vi "LVIS_FilePosition.vi"(8 "Error In":errorcluster, 9 "Action":enum16{"Read", "Write", "Set"}(ring), 10 "Position In":i32, 11 "Ref In":refnum<file>) -> (0 "Error out":errorcluster, 2 "Position Out":i32, 3 "Ref Out":refnum<file>)   [LabVIEW 2015]
doc: "Reads, writes and sets the current backup file position based on the LVIS_Setting FilePosition value."
uses:
  Globals/LVIS_IsGlobal.vi
  <vilib>/Utility/config.llb/Read Key (String).vi
  <vilib>/Utility/config.llb/Write Key (String).vi
  <vilib>/Utility/config.llb/NI_LVConfig.lvlib
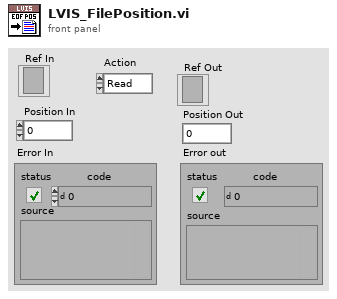
[diagram p1: front panel]
types:
  T1 = typedef "NI_LVConfig.lvlib/Config Data RefNum.ctl" = refnum<k1>
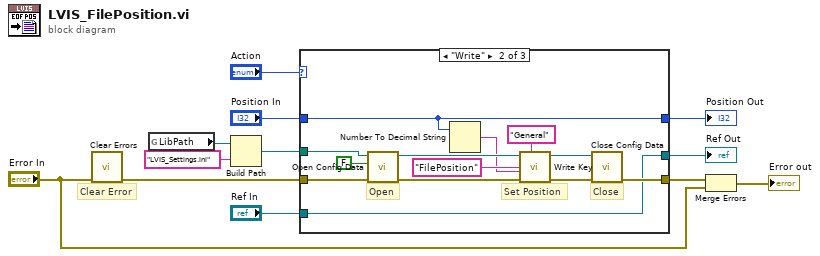
[diagram p0: block diagram]
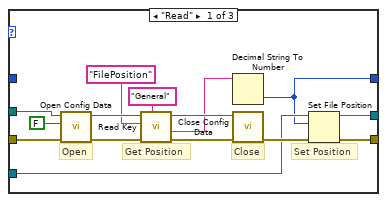
[diagram p2: hidden frame]
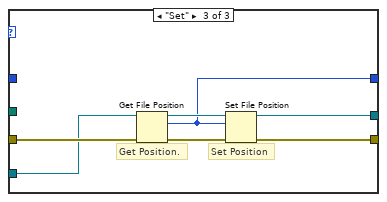
[diagram p3: hidden frame]
diagram:
  # "Clear Error"
  n1 = call <vilib>:"Clear Errors.vi"("error in (no error)"="Error In") -> ("error out"=w7:errorcluster)  [unwired: 5 in, 1 out]
  n2 = global read "LVIS_IsGlobal.vi" "LibPath"() -> (w3:path)
  n3 = Build Path(base path=w3, name or relative path="LVIS_Settings.ini") -> (appended path=w1:path)
  n4 = case shown="\"Write\"" "Action" {
    tunnel: w7 -> [w27 w40 w45]
    tunnel: [w14 w32 w44] -> w6
    tunnel: w1 -> [w18 w30 _]
    tunnel: "Position In" -> [_ w28 _]
    tunnel: "Ref In" -> [w16 w29 w43]
    tunnel: [w15 w29 w42] -> w9
    tunnel: [w13 w28 w41] -> w8
    frame "Read" {
      # "Set Position"
      # "Close"
      # "Get Position"
      # "Open"
      n5 = call <vilib>:"Open Config Data.vi"("error in (no error)"=w27, "create file if necessary (T)"=FALSE, "configuration file path"=w18) -> ("error out"=w25:errorcluster, "refnum"=w24:T1)  [unwired: 6 in, 1 out]
      n6 = call-poly <vilib>:"Read Key.vi"("section"="General", "error in (no error)"=w25, "key"="FilePosition", "refnum"=w24) -> ("error out"=w21:errorcluster, "value"=w19:string, "refnum out"=w20:T1)  [unwired: 4 in, 1 out]
      n7 = Decimal String To Number(string=w19) -> (number=w13:i32)  [unwired: 2 in, 1 out]
      n8 = call <vilib>:"Close Config Data.vi"("error in (no error)"=w21, "refnum"=w20) -> ("error out"=w17:errorcluster)  [unwired: 8 in, 1 out]
      n9 = Set File Position(offset (in bytes) (0)=w13, refnum=w16, error in=w17) -> (refnum out=w15:refnum<file>, error out=w14:errorcluster)  [unwired: 1 in]
    }
    frame "Write" {
      # "Close"
      # "Set Position"
      # "Open"
      n10 = call <vilib>:"Open Config Data.vi"("error in (no error)"=w40, "create file if necessary (T)"=FALSE, "configuration file path"=w30) -> ("error out"=w38:errorcluster, "refnum"=w37:T1)  [unwired: 6 in, 1 out]
      n11 = Number To Decimal String(number=w28) -> (decimal integer string=w31:string)  [unwired: 1 in]
      n12 = call-poly <vilib>:"Write Key.vi"("section"="General", "error in (no error)"=w38, "value"=w31, "key"="FilePosition", "refnum"=w37) -> ("error out"=w34:errorcluster, "refnum out"=w33:T1)  [unwired: 4 in, 1 out]
      n13 = call <vilib>:"Close Config Data.vi"("error in (no error)"=w34, "refnum"=w33) -> ("error out"=w32:errorcluster)  [unwired: 8 in, 1 out]
    }
    frame "Set" {
      # "Set Position"
      # "Get Position."
      n14 = Get File Position(4:w45, 7:w43) -> (0:w47:errorcluster, 2:w41:i64, 3:w46:refnum<file>)
      n15 = Set File Position(offset (in bytes) (0)=w41, refnum=w46, error in=w47) -> (refnum out=w42:refnum<file>, error out=w44:errorcluster)  [unwired: 1 in]
    }
  }
  "Ref Out" <- w9
  "Position Out" <- w8
  n16 = Merge Errors(w6, "Error In") -> (→"Error out":errorcluster)
